vi "SUB_TestSound_NewFormat.vi"(0 "Test Item":string, 1 "SPEC Max Sound Level":dbl, 3 "Sending Ao Name":string, 5 "Test Freq(HZ)":string, 9 "SPEC TXRX Diff HZ":dbl, 11 "SPEC Min Sound Level":dbl, 12 "SPEC THD %":dbl, 13 "Receiving Ai Name":string, 14 "Ao Voltage":dbl) -> (4 "output cluster":T1)   [LabVIEW 2011]
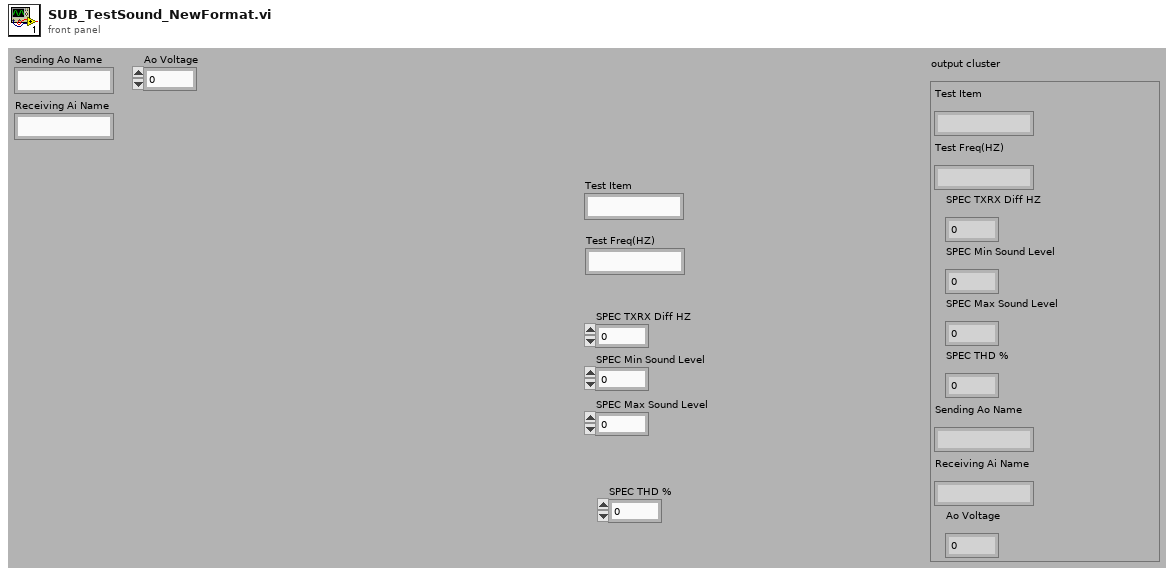
[diagram p1: front panel]
types:
  T1 = cluster{"Test Item":string, "Test Freq(HZ)":string, "SPEC TXRX Diff HZ":dbl, "SPEC Min Sound Level":dbl, "SPEC Max Sound Level":dbl, "SPEC THD %":dbl, "Sending Ao Name":string, "Receiving Ai Name":string, "Ao Voltage":dbl}
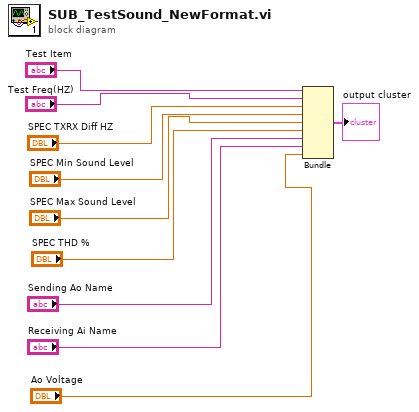
[diagram p0: block diagram]
diagram:
  n1 = Bundle("Test Item"="Test Item", "Test Freq(HZ)"="Test Freq(HZ)", "SPEC TXRX Diff HZ"="SPEC TXRX Diff HZ", "SPEC Min Sound Level"="SPEC Min Sound Level", "SPEC Max Sound Level"="SPEC Max Sound Level", "SPEC THD %"="SPEC THD %", "Sending Ao Name"="Sending Ao Name", "Receiving Ai Name"="Receiving Ai Name", "Ao Voltage"="Ao Voltage") -> (→"output cluster":T1)  [unwired: 1 in]
